vi "Set Group Properties.vi"(5 "Group Description":string, 7 "Group Name":string, 8 "error in (no error)":errorcluster, 10 "Channel Names + Properties":string[][](array[string]), 11 "TDMS in":refnum<class "TDMS.lvclass">) -> (0 "error out":errorcluster, 3 "TDMS out":refnum<class "TDMS.lvclass">)   [LabVIEW 2017, in "Report_lib.lvlib" / "TDMS.lvclass"]
doc: "Write Group and Channels properties\nas 2d STR array"
uses:
  TDMS.lvclass
  TDMS.lvclass/TDMS.ctl
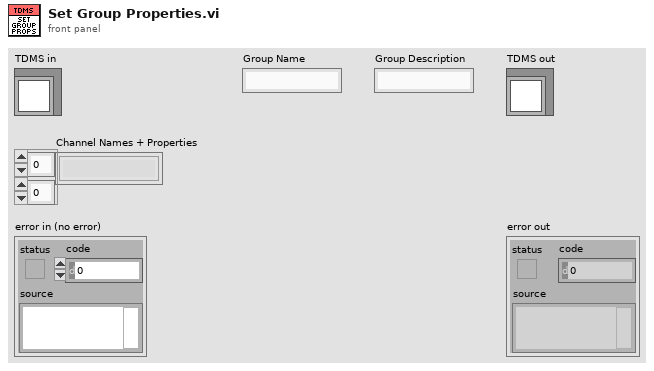
[diagram p1: front panel]
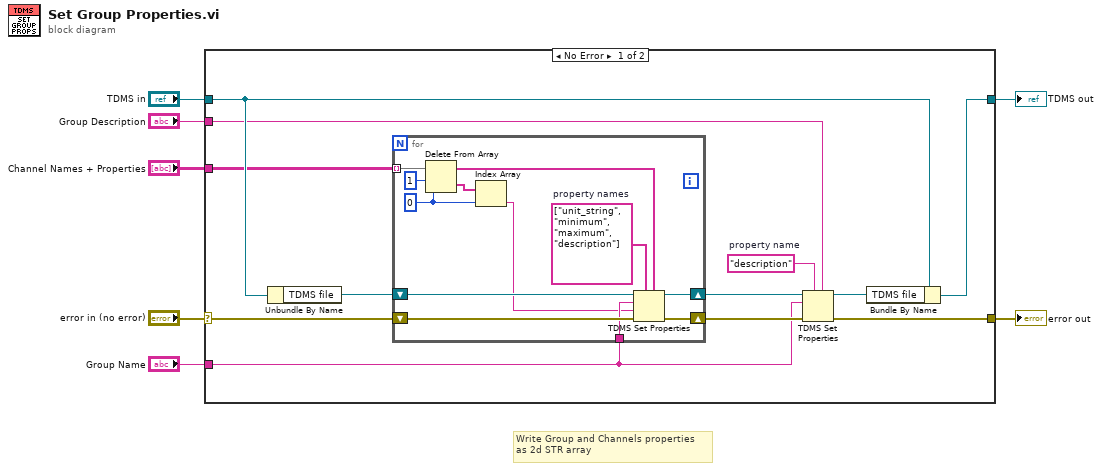
[diagram p0: block diagram]
diagram:
  # "Write Group and Channels properties\nas 2d STR array"
  n1 = case shown="No Error" "error in (no error)" {
    selector: "error in (no error)" -> [w14 w33]
    tunnel: [w13 w33] -> w6
    tunnel: [w18 w32] -> w4
    tunnel: "TDMS in" -> [w19 w32]
    tunnel: "Group Name" -> [w10 _]
    tunnel: "Group Description" -> [w9 _]
    tunnel: "Channel Names + Properties" -> [w8 _]
    frame No Error {
      w17 = "description"  # property name
      n2 = Unbundle By Name(w19) -> ("TDMS file"=w11:refnum<k34>)
      n3 = for {
        shift-right: [w29] -> w15
        shift-left: w11 -> [w31]
        shift-right: [w28] -> w16
        shift-left: w14 -> [w30]
        tunnel: w10 -> [w26]
        tunnel: w8 -> [w25] mode=indexing
        w21 = 0 ("index")
        w27 = string[] ["unit_string", "minimum", "maximum", "description"]  # property names
        n4 = Delete From Array(array=w25, length=1, index=w21) -> (deleted portion=w22:string[], array with subset deleted=w23:string[])
        n5 = Index Array(array=w22, index=w21) -> (element=w20:string)
        n6 = TDMS Set Properties(5:w23, 7:w27, 8:w30, 9:w20, 10:w26, 11:w31) -> (0:w28:errorcluster, 3:w29:refnum<k34>)  [unwired: 2 out]
      }
      n7 = TDMS Set Properties(5:w9, 7:w17, 8:w16, 10:w10, 11:w15) -> (0:w13:errorcluster, 3:w12:refnum<k34>)  [unwired: 1 in, 2 out]
      n8 = Bundle By Name(cluster=w19, "TDMS file"=w12) -> (w18:refnum<class "TDMS.lvclass">)
    }
    frame Error {
    }
  }
  "error out" <- w6
  "TDMS out" <- w4
